vi "ConfigStartCards.vi"(4 "Sample Clock Export":T2, 5 "Error In":errorcluster, 6 "Reference Clock Properties":T3={"RefClockGlobalName"="/PXI1Slot2/10MHzRefClock", "RefClockRate"=10000000.0}, 7 "DAQ Setup Array":T4[](array[typedef]) {"Configuration" items=["Differential"=10106, "RSE"=10083, "NRSE"=10078, "Pseudodifferential"=12529]}, 8 "General HardWare Constants":T1={"Nr. of Columns"=15, "Nr. of Rows"=15, "OverSampling"=2, "Fetch Rate "=10, "Sampling Rate"=0, "Nr. of BNC inputs"=3, "Sample Strip Length"=10}) -> (0 "error out":errorcluster, 1 "Sample Clock":tag[](array[tag]), 2 "Start Edge":tag, 3 "Tasks Out":refnum<k21>[](array[refnum]))   [LabVIEW 2012]
uses:
  controls/DAQ Setup.ctl
  controls/RefClockSettings.ctl
  controls/SampleClockExport.ctl
  controls/General Hardware config.ctl
  <vilib>/DAQmx/create/channels.llb/DAQmx Create Channel (AI-Voltage-Basic).vi
  <vilib>/DAQmx/configure/timing.llb/DAQmx Timing (Sample Clock).vi
  <vilib>/DAQmx/configure/events/hardwareSignals.llb/DAQmx Export Signal (Most Signals).vi
  <vilib>/DAQmx/configure/trigger.llb/DAQmx Start Trigger (Digital Edge).vi
  <resource>/objmgr/daqmx.rc
panel:
  out "Array 2":bool[](array[boolean])
  out "Devices":tag[][](array[tag])
  out "Array":string[](array[string])
  # "Array"
  # "Acq. System"
  # "Other analog Input"
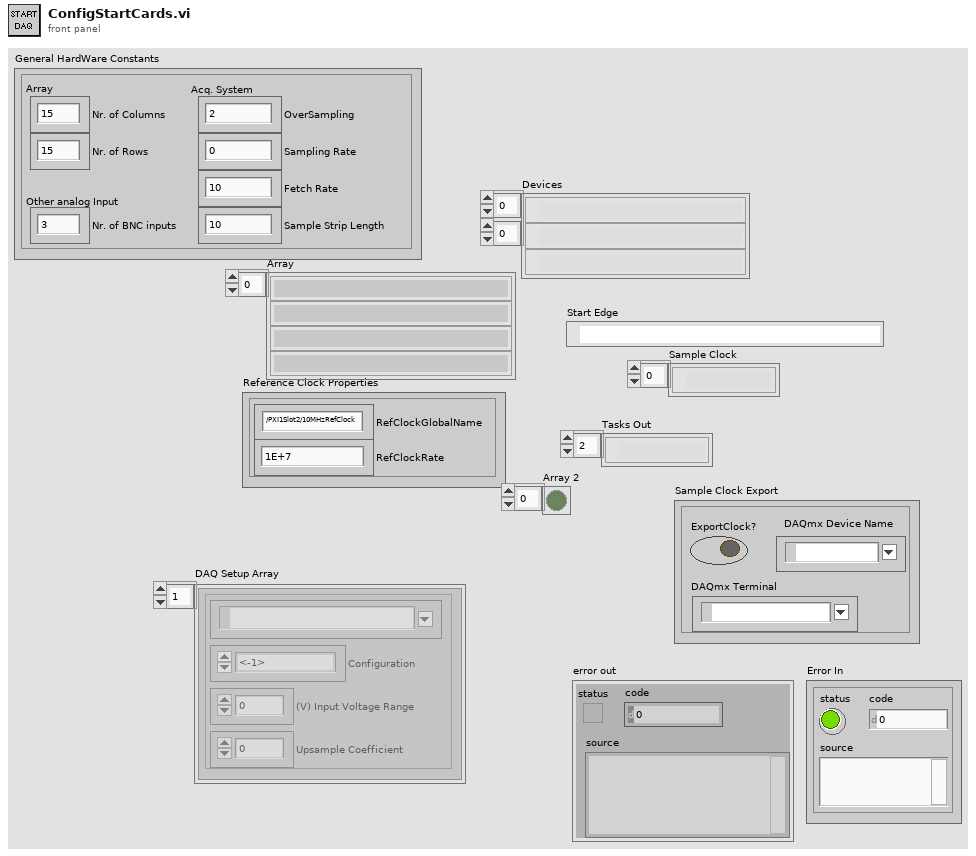
[diagram p1: front panel]
types:
  T1 = typedef "General Hardware config.ctl" = cluster{"Nr. of Columns":i32, "Nr. of Rows":i32, "OverSampling":i32, "Fetch Rate ":i32, "Sampling Rate":i32, "Nr. of BNC inputs":i32, "Sample Strip Length":i32}
  T2 = typedef "SampleClockExport.ctl" = cluster{"DAQmx Terminal":tag, "ExportClock?":bool, "DAQmx Device Name":tag}
  T3 = typedef "RefClockSettings.ctl" = cluster{"RefClockGlobalName":string, "RefClockRate":dbl}
  T4 = typedef "DAQ Setup.ctl" = cluster{"Input Voltage Range":dbl, "Upsample Coefficient":u32, "Analog Input Channels":tag, "Configuration":i32}
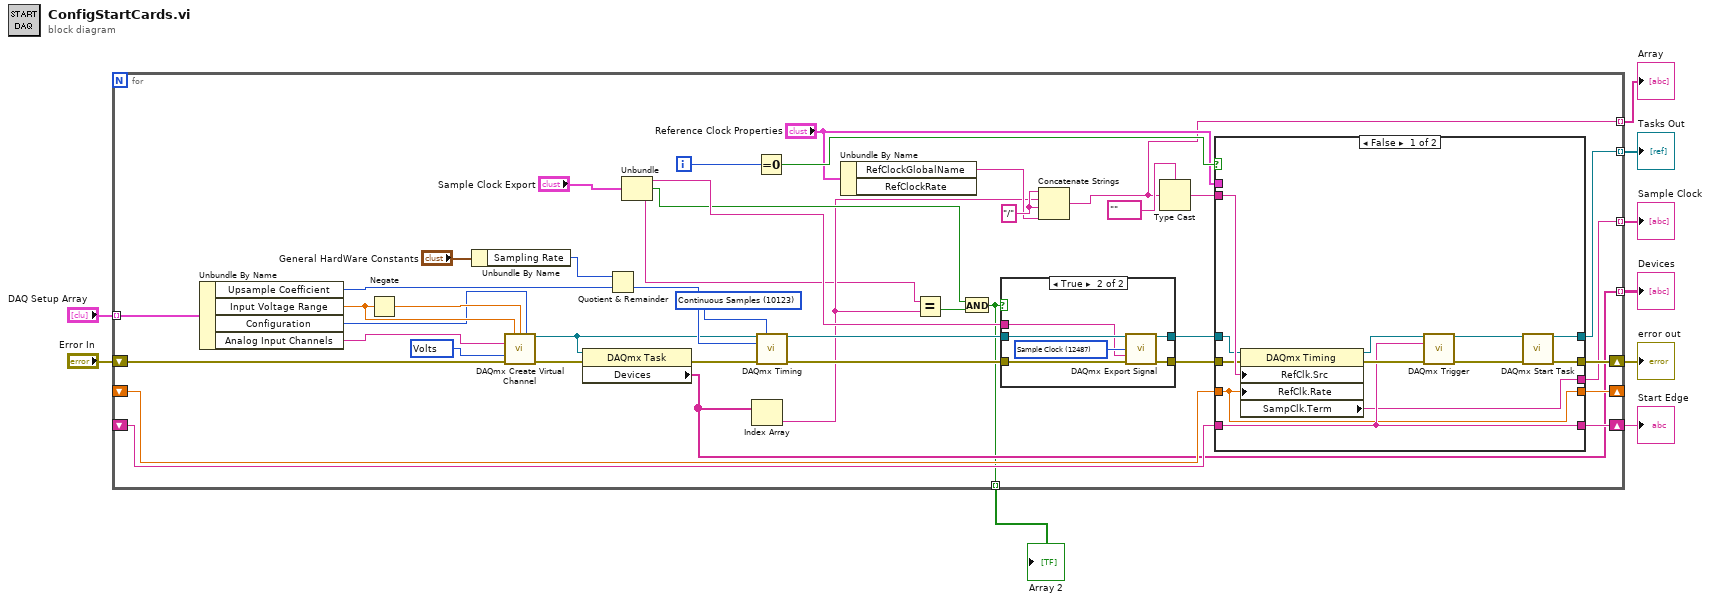
[diagram p0: block diagram]
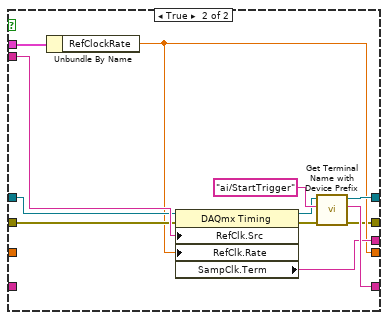
[diagram p3: hidden frame]
diagram:
  n1 = for {
    tunnel: "DAQ Setup Array" -> [w51] mode=indexing
    shift-right: [w43] -> w8
    shift-left: "Error In" -> [w39]
    shift-right: [w45] -> _
    shift-left: _ -> [w42]
    shift-right: [w44] -> w6
    shift-left: _ -> [w41]
    tunnel: [w40] -> w7 mode=indexing
    tunnel: [w36] -> w4 mode=indexing
    tunnel: [w23] -> w3 mode=indexing
    tunnel: [w20] -> w2 mode=indexing
    tunnel: [w10] -> w1 mode=indexing
    i -> [w29]
    w18 = "/"
    w47 = 10123 items=["Finite Samples"=10178, "Continuous Samples"=10123, "Hardware Timed Single Point"=12522] ("sample mode")
    w48 = 10348 items=["Volts"=10348, "From Custom Scale"=10065] ("units")
    n2 = Unbundle By Name(w51) -> ("Upsample Coefficient"=w38:u32, "Input Voltage Range"=w49:dbl, "Configuration"=w19:i32, "Analog Input Channels"=w27:tag)
    n3 = Negate(x=w49) -> (-x=w50:dbl)
    n4 = Unbundle By Name("General HardWare Constants") -> ("Sampling Rate"=w15:i32)
    n5 = call-poly <vilib>:"DAQmx Create Virtual Channel.vi"("maximum value"=w49, "minimum value"=w50, "input terminal configuration"=w19, "physical channels"=w27, "units"=w48, "error in"=w39) -> ("task out"=w26:refnum<k21>, "error out"=w22:errorcluster)  [unwired: 8 in]
    n6 = property class="DAQmx Task"(reference=w26, error in=w22) -> (error out=w21:errorcluster, "Devices"=w20:tag[])  [unwired: 1 out]
    n7 = Quotient & Remainder(x=w15, y=w38) -> (floor(x/y)=w37:u32)  [unwired: 1 out]
    n8 = Unbundle("Sample Clock Export") -> ("DAQmx Terminal"=w28:tag, "ExportClock?"=w14:bool, "DAQmx Device Name"=w11:tag)
    n9 = Index Array(array=w20) -> (element=w12:tag)  [unwired: 1 in]
    n10 = Equal To 0?(x=w29) -> (x = 0?=w46:bool)
    n11 = call-poly <vilib>:"DAQmx Timing.vi"("task/channels in"=w26, "sample mode"=w47, "rate"=w37, "error in"=w21) -> ("task out"=w32:refnum<k21>, "error out"=w34:errorcluster)  [unwired: 10 in]
    n12 = Unbundle By Name("Reference Clock Properties") -> ("RefClockGlobalName"=w17:string)  [unwired: 1 out]
    n13 = Equal?(x=w11, y=w12) -> (x = y?=w13:bool)
    n14 = And(x=w14, y=w13) -> (x .and. y?=w10:bool)
    n15 = case shown="True" w10 {
      tunnel: w34 -> [w53 w58]
      tunnel: [w53 w57] -> w33
      tunnel: w32 -> [w52 w55]
      tunnel: [w52 w56] -> w31
      tunnel: w28 -> [_ w54]
      frame False {
      }
      frame True {
        w59 = 12487 items=["AI Convert Clock"=12484, "10MHz Reference Clock"=12536, "20MHz Timebase Clock"=12486, "Sample Clock"=12487, "Advance Trigger"=12488, "Reference Trigger"=12490, "Start Trigger"=12491, "Advance Complete Event"=12492, "AI Hold Complete Event"=12493, "Counter Output Event"=12494, "Change Detection Event"=12511, "Watchdog Timer Expired Event"=12512] ("signal")
        n16 = call-poly <vilib>:"DAQmx Export Signal.vi"("task/channels in"=w55, "signal"=w59, "output terminal"=w54, "error in"=w58) -> ("task out"=w56:refnum<k21>, "error out"=w57:errorcluster)  [unwired: 10 in]
      }
    }
    n17 = Concatenate Strings(w18, w12, w18, w17) -> (w23:string)
    n18 = Type Cast(type=tag "", x=w23) -> (*(type *) &x=w25:tag)
    n19 = case shown="False" w46 {
      tunnel: w31 -> [w67 w74]
      tunnel: w25 -> [w71 w83]
      tunnel: [w68 w73] -> w45
      tunnel: [w69 w81] -> w44
      tunnel: [w64 w72] -> w43
      tunnel: w42 -> [w68 _]
      tunnel: w41 -> [w69 _]
      tunnel: [w63 w80] -> w40
      tunnel: w33 -> [w66 w79]
      tunnel: [w61 w76] -> w36
      tunnel: "Reference Clock Properties" -> [_ w75]
      frame False {
        n20 = property class="DAQmx Timing"(reference=w67, error in=w66, "RefClk.Src"=w71, "RefClk.Rate"=w68) -> (reference out=w60:refnum<k21>, error out=w70:errorcluster, "SampClk.Term"=w61:tag)
        n21 = call-poly <vilib>:"DAQmx Trigger.vi"("task/channels in"=w60, "source"=w69, "error in"=w70) -> ("task out"=w62:refnum<k21>, "error out"=w65:errorcluster)  [unwired: 11 in]
        n22 = call <vilib>:"DAQmx Start Task.vi"("task/channels in"=w62, "error in"=w65) -> ("task out"=w63:refnum<k21>, "error out"=w64:errorcluster)  [unwired: 12 in]
      }
      frame True {
        n23 = Unbundle By Name(w75) -> ("RefClockRate"=w73:dbl)
        n24 = property class="DAQmx Timing"(reference=w74, error in=w79, "RefClk.Src"=w83, "RefClk.Rate"=w73) -> (reference out=w77:refnum<k21>, error out=w78:errorcluster, "SampClk.Term"=w76:tag)
        n25 = call "Get Terminal Name with Device Prefix.vi"("error in (no error)"=w78, "Local Terminal Name"="ai/StartTrigger", "task/channels in"=w77) -> ("error out"=w72:errorcluster, "Terminal Name with Device Prefix"=w81:tag, "task out"=w80:refnum<k21>)  [unwired: 6 in]
      }
    }
  }
  "error out" <- w8
  "Tasks Out" <- w7
  "Start Edge" <- w6
  "Sample Clock" <- w4
  "Array" <- w3
  "Devices" <- w2
  "Array 2" <- w1
